vi "_dbmgr_thread.vi"(8 "Error in":errorcluster caption="Error in (no error)", 11 "SyncQ":refnum<queue>) -> (0 "Error out":errorcluster)   [LabVIEW 2017, in "TagDB.lvlib"]
uses:
  TagDB.lvlib
  _db.vi
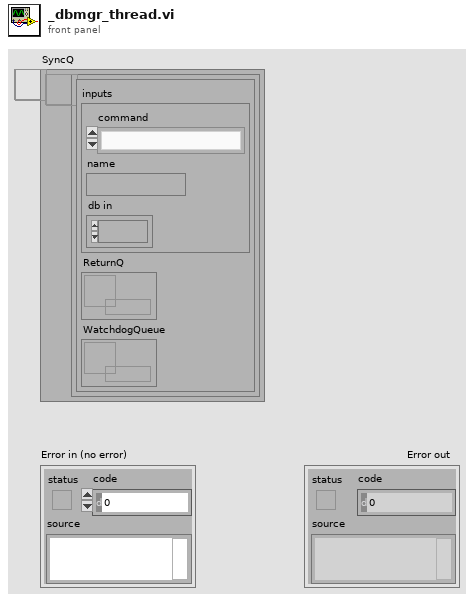
[diagram p1: front panel]
types:
  T1 = cluster{"inputs":cluster{"command":enum16{"create", "destroy", "cleanUp", "list", "get info", "force destroy"}, "name":string, "db in":refnum<k1>}, "ReturnQ":refnum<queue>, "WatchdogQueue":refnum<queue>}
  T2 = cluster{"command":enum16{"create", "destroy", "cleanUp", "list", "get info", "force destroy"}, "name":string, "db in":refnum<k1>}
  T3 = enum16{"create", "destroy", "cleanUp", "list", "get info", "force destroy"}
  T4 = cluster{"db out":refnum<k1>, "db list":string[], "info":cluster{"db":refnum<k1>, "Count":i32}, "created new?":bool, "error out":errorcluster}
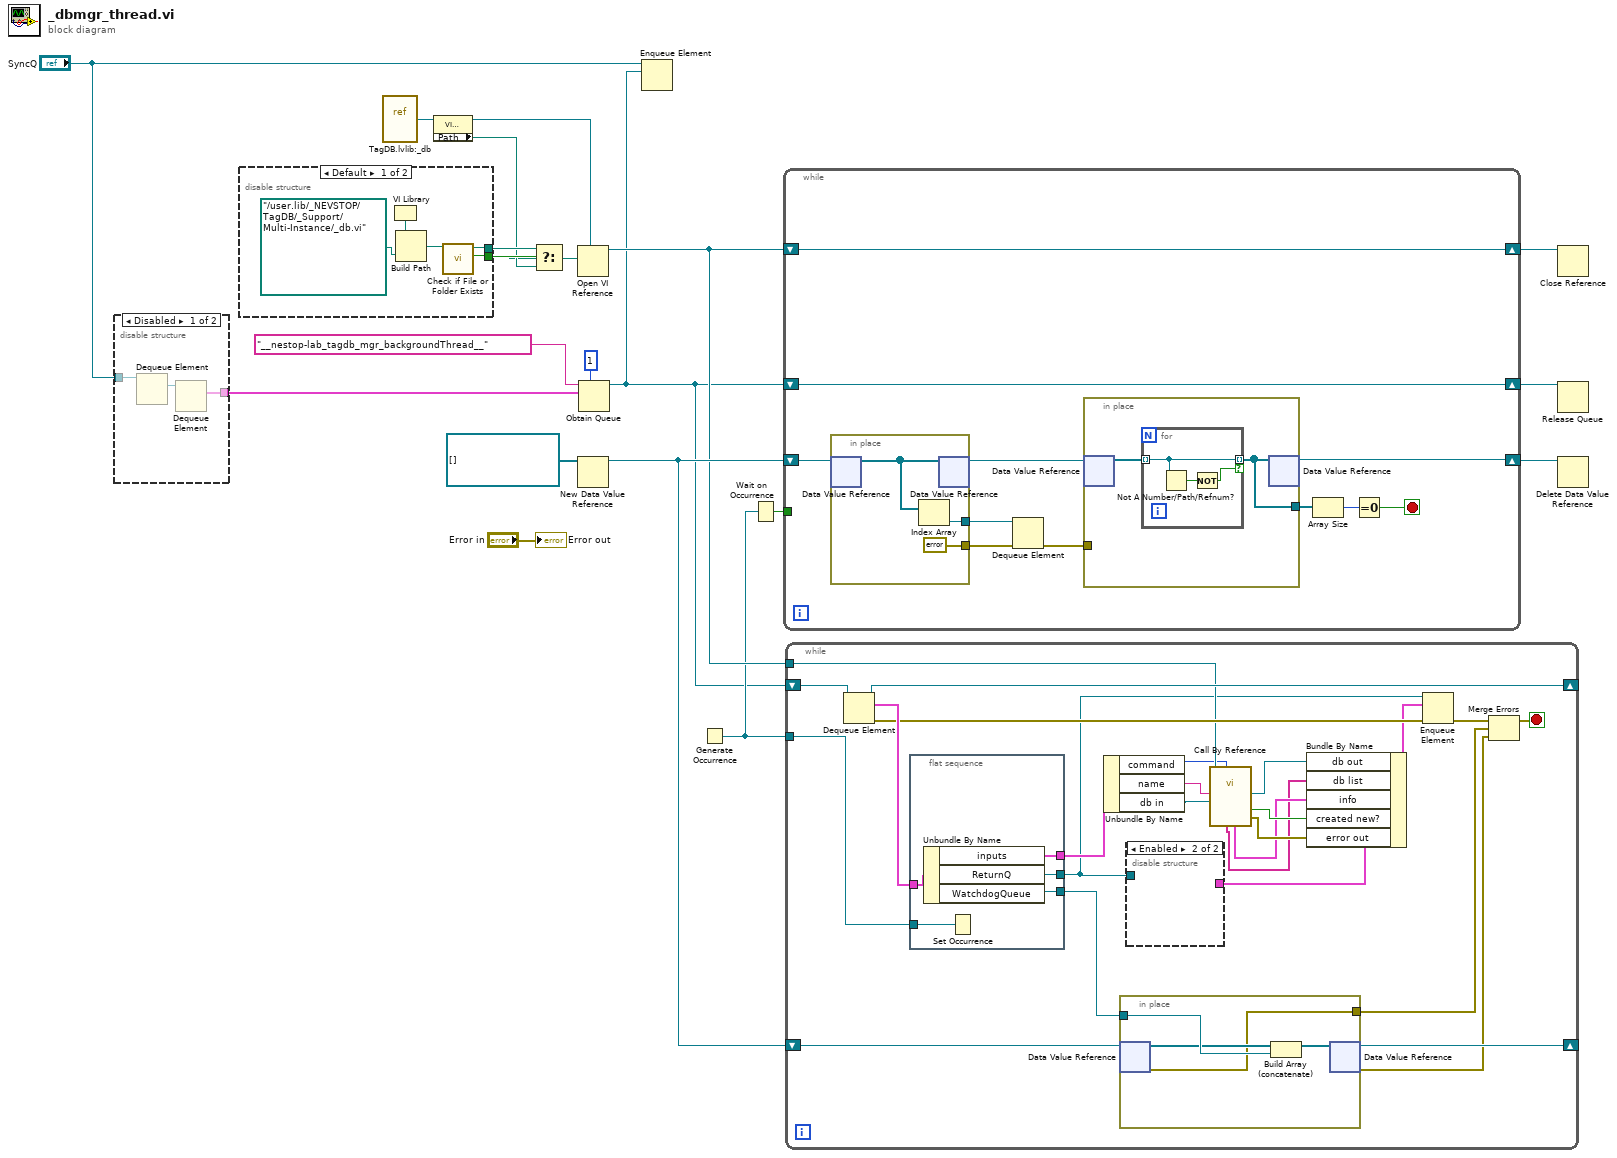
[diagram p0: block diagram]
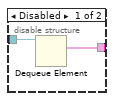
[diagram p2: hidden frame]
diagram:
  n1 = disable-structure shown="Disabled" {
    disable-tunnel: "SyncQ" -> [w23 _]
    disable-tunnel: [w21 _] -> w1
    frame Disabled {
      n2 = Dequeue Element(queue=w23) -> (element=w22:refnum<queue>)  [unwired: 2 in, 3 out]
      n3 = Dequeue Element(queue=w22) -> (element=w21:T1)  [unwired: 2 in, 3 out]
    }
    frame Enabled {
    }
  }
  n4 = disable-structure shown="Default" {
    disable-tunnel: [w24 _] -> w10
    disable-tunnel: [w25 _] -> w9
    frame condition #0 (active) {
      n5 = VI Library() -> (path=w28:path)
      n6 = Build Path(base path=w28, name or relative path=path "../user.lib/_NEVSTOP/TagDB/_Support/Multi-Instance/_db.vi" ("Relative path (.)")) -> (appended path=w27:path)
      n7 = call <vilib>:"Check if File or Folder Exists.vi"("path"=w27) -> ("file or folder exists?"=w24:bool, "dup path"=w25:path)  [unwired: 8 in, 1 out]
    }
    frame condition #1 {
    }
  }
  n8 = vi-ref "TagDB.lvlib:_db.vi"() -> (w20:refnum<vi>)
  n9 = property class="VI (strict)"(reference=w20) -> (reference out=w19:refnum<vi>, "Path"=w8:path)  [unwired: 1 in, 1 out]
  n10 = Select(t=w9, s=w10, f=w8) -> (s? t:f=w7:path)
  n11 = Open VI Reference(type specifier VI Refnum (for type only)=w19, vi path=w7) -> (vi reference=w12:refnum<vi>)  [unwired: 4 in, 1 out]
  n12 = New Data Value Reference(data value=refnum<queue>[] [] ("WatchdogQueue")) -> (data value reference=w17:refnum<data-value>)  [unwired: 1 in, 1 out]
  n13 = Obtain Queue(max queue size (-1, unlimited)=1, name (unnamed)="__nestop-lab_tagdb_mgr_backgroundThread__", element data type=w1) -> (queue out=w3:refnum<queue>)  [unwired: 2 in, 2 out]
  n14 = Enqueue Element(queue="SyncQ", element=w3) -> ()  [unwired: 2 in, 3 out]
  n15 = Generate Occurrence() -> (w5:refnum<k4>)
  n16 = Wait on Occurrence(2:w5) -> (0:w4:bool)  [unwired: 2 in]
  n17 = while {
    shift-right: [w33] -> w16
    shift-left: w17 -> [w39]
    shift-right: [w31] -> w15
    shift-left: w3 -> [w31]
    shift-right: [w32] -> w14
    shift-left: w12 -> [w32]
    tunnel: w4 -> [_]
    stop <- w29 stop-if-true
    n18 = in-place {
      in-place-border: [w46] -> w38
      in-place-border: [errorcluster {"status"=FALSE, "code"=0, "source"=""} ("error in (no error)")] -> w36
      n19 = in-place-dvr #1(w39) -> (w47:refnum<queue>[])  [unwired: 1 out]
      n20 = Index Array(array=w47) -> (element=w46:refnum<queue>)  [unwired: 1 in]
      n21 = in-place-dvr #1(w47) -> (w37:refnum<data-value>)  [unwired: 1 out]
    }
    n22 = Dequeue Element(queue=w38, error in (no error)=w36) -> (error out=w35:errorcluster)  [unwired: 1 in, 3 out]
    n23 = in-place {
      in-place-border: w35 -> [_]
      in-place-border: [w40] -> w34
      n24 = in-place-dvr #2(w37) -> (w41:refnum<queue>[])  [unwired: 1 out]
      n25 = for {
        tunnel: w41 -> [w43] mode=indexing
        tunnel: [w43] -> w40 mode=indexing if=w42
        n26 = Not A Number/Path/Refnum?(number/path/refnum=w43) -> (NaN/Path/Refnum?=w44:bool)
        n27 = Not(x=w44) -> (.not. x?=w42:bool)
      }
      n28 = in-place-dvr #2(w40) -> (w33:refnum<data-value>)  [unwired: 1 out]
    }
    n29 = Array Size(array=w34) -> (size(s)=w30:i32)
    n30 = Equal To 0?(x=w30) -> (x = 0?=w29:bool)
  }
  n31 = while {
    shift-right: [w67] -> _
    shift-left: w17 -> [w68]
    shift-right: [w69] -> _
    shift-left: w3 -> [w72]
    tunnel: w12 -> [w60]
    tunnel: w5 -> [w61]
    stop <- w65 stop-if-true
    n32 = Dequeue Element(queue=w72) -> (queue out=w69:refnum<queue>, element=w71:T1, error out=w66:errorcluster)  [unwired: 2 in, 1 out]
    n33 = flat-sequence {
      tunnel: w71 -> [w79]
      tunnel: [w78] -> w70
      tunnel: [w77] -> w55
      tunnel: w61 -> [w76]
      tunnel: [w75] -> w59
      frame #0 {
        n34 = Unbundle By Name(w79) -> ("inputs"=w75:T2, "ReturnQ"=w77:refnum<queue>, "WatchdogQueue"=w78:refnum<queue>)
        n35 = Set Occurrence(w76) -> ()
      }
    }
    n36 = Unbundle By Name(w59) -> ("command"=w58:T3, "name"=w57:string, "db in"=w56:refnum<k1>)
    n37 = in-place {
      in-place-border: w70 -> [w83]
      in-place-border: [w80] -> w62
      n38 = in-place-dvr #3(w68) -> (w82:refnum<queue>[], w80:errorcluster)
      n39 = Build Array (concatenate)(w82, w83) -> (w81:refnum<queue>[])
      n40 = in-place-dvr #3(w81) -> (w67:refnum<data-value>, w64:errorcluster)
    }
    n41 = disable-structure shown="Enabled" {
      disable-tunnel: w55 -> [w74 _]
      disable-tunnel: [w73 _] -> w54
      frame Disabled {
        n42 = Dequeue Element(queue=w74) -> (element=w73:T4)  [unwired: 2 in, 3 out]
      }
      frame Enabled {
      }
    }
    n43 = call-by-ref "?"(reference=w60, "command"=w58, "db in"=w56, "name"=w57) -> ("error out"=w50:errorcluster, "created new?"=w51:bool, "db out"=w52:refnum<k1>, "info"=w49:cluster{"db":refnum<k1>, "Count":i32}, "db list"=w48:string[])  [unwired: 5 in, 2 out]
    n44 = Bundle By Name(cluster=w54, "db out"=w52, "db list"=w48, "info"=w49, "created new?"=w51, "error out"=w50) -> (w53:T4)
    n45 = Enqueue Element(queue=w55, element=w53, error in (no error)=w66) -> (error out=w63:errorcluster)  [unwired: 1 in, 2 out]
    n46 = Merge Errors(w63, w62, w64) -> (w65:errorcluster)
  }
  n47 = Close Reference(reference=w14) -> ()  [unwired: 1 in, 1 out]
  n48 = Release Queue(queue=w15) -> ()  [unwired: 2 in, 3 out]
  n49 = Delete Data Value Reference(data value reference=w16) -> ()  [unwired: 1 in, 2 out]
  "Error out" <- "Error in"
